vi "程序下载-V1.0.1.vi"() -> ()   [LabVIEW 2013]
uses:
  SxsenderClassLibrary.dll
panel:
  out "x/y":dbl format="%.1f"
  in  "SX文件路径 2":path
  in  "基路径 2":path=path "C:/Program Files/National Instruments/LabVIEW 2013/temp"
  out "添加的路径":path
  out "引用输出":refnum<k24>
  in  "布尔":bool
  in  "停止":bool
  in  "基路径":path=path "C:/Program Files/National Instruments/LabVIEW 2013/temp"
  out "错误输出":errorcluster
  in  "停止":bool
  out "字符串":string
  in  "结果":i32(listbox)=-1
  out "Schedule":u8(slide) scale=0.0..100.0
  in  "Slave NO.":u16(ring) items=["1", "2", "3", "4", "5", "6", "7", "8", "9", "10", "11", "12", "13", "14", "15", "16", "17", "18", "19", "20", "21", "22", "23", "24", "25", "26", "27", "28", "29", "30", ""]
  in  "CAN端口 2":u16(ring)=2 caption="TargetBoard" items=["BCU"=1, "BMU"=2]
  in  "波特率":u16(ring)=500 caption="Baudrate" items=["5Kbps"=5, "10Kbps"=10, "20Kbps"=20, "40Kbps"=40, "50Kbps"=50, "80Kbps"=80, "100Kbps"=100, "125Kbps"=125, "200Kbps"=200, "250Kbps"=250, "400Kbps"=400, "500Kbps"=500, "666Kbps"=666, "800Kbps"=800, "1000Kbps"=1000]
  in  "STOP":bool
  in  "Continue":bool
  in  "START":bool
  in  "SX File Path":path
  in  "CAN端口":u16(ring) caption="CANIndex" items=["0", "1"]
  in  "CAN卡类型":u32(ring)=4 caption="DevType" items=["PCI5121"=1, "PCI9810"=2, "USBCAN1"=3, "USBCAN2"=4, "PCI9820"=5, "PCI5110"=7, "CANLite(mini)"=8, "ISA9620"=9, "ISA5420"=10, "PC104CAN"=11, "DNP9810"=13, "PCI9840B"=14, "PC104C2"=15, "PCI9820I"=16, "pec9920"=18, "USBCAN_E_U"=20, "USBCAN_2E_U"=21]
  in  "设备索引号":u16(ring) caption="DevIndex" items=["0", "1", "2", "3", "4", "5", "6", "7", "8", "9", "10", "11", "12", "13", "14", "15", "16"]
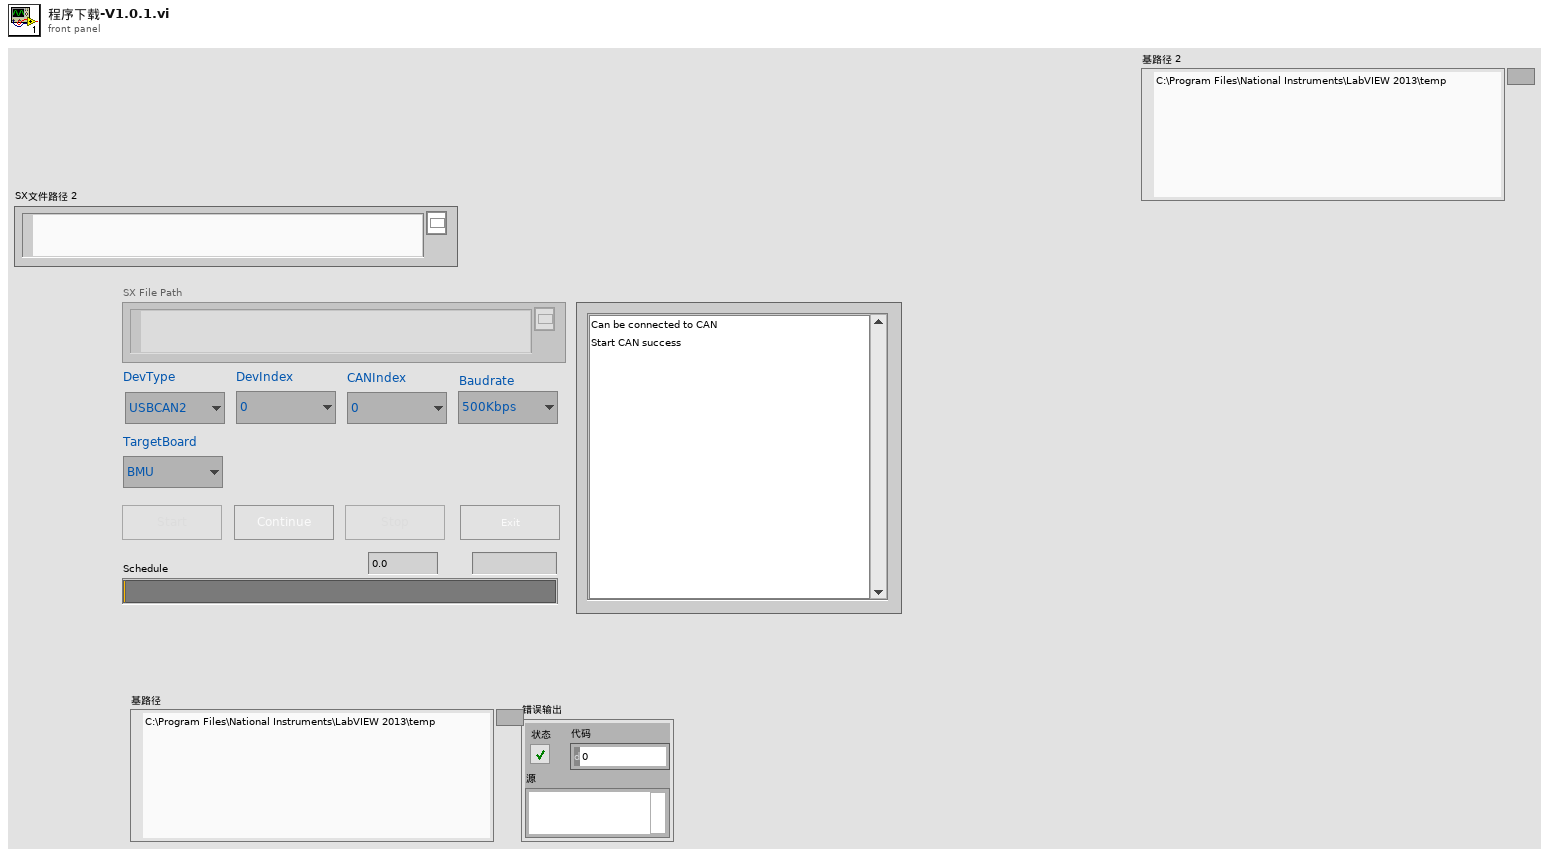
[diagram p1: front panel]
types:
  T1 = enum32{"Invalid", "Standard", "Closed", "Hidden", "Minimized", "Maximized"}
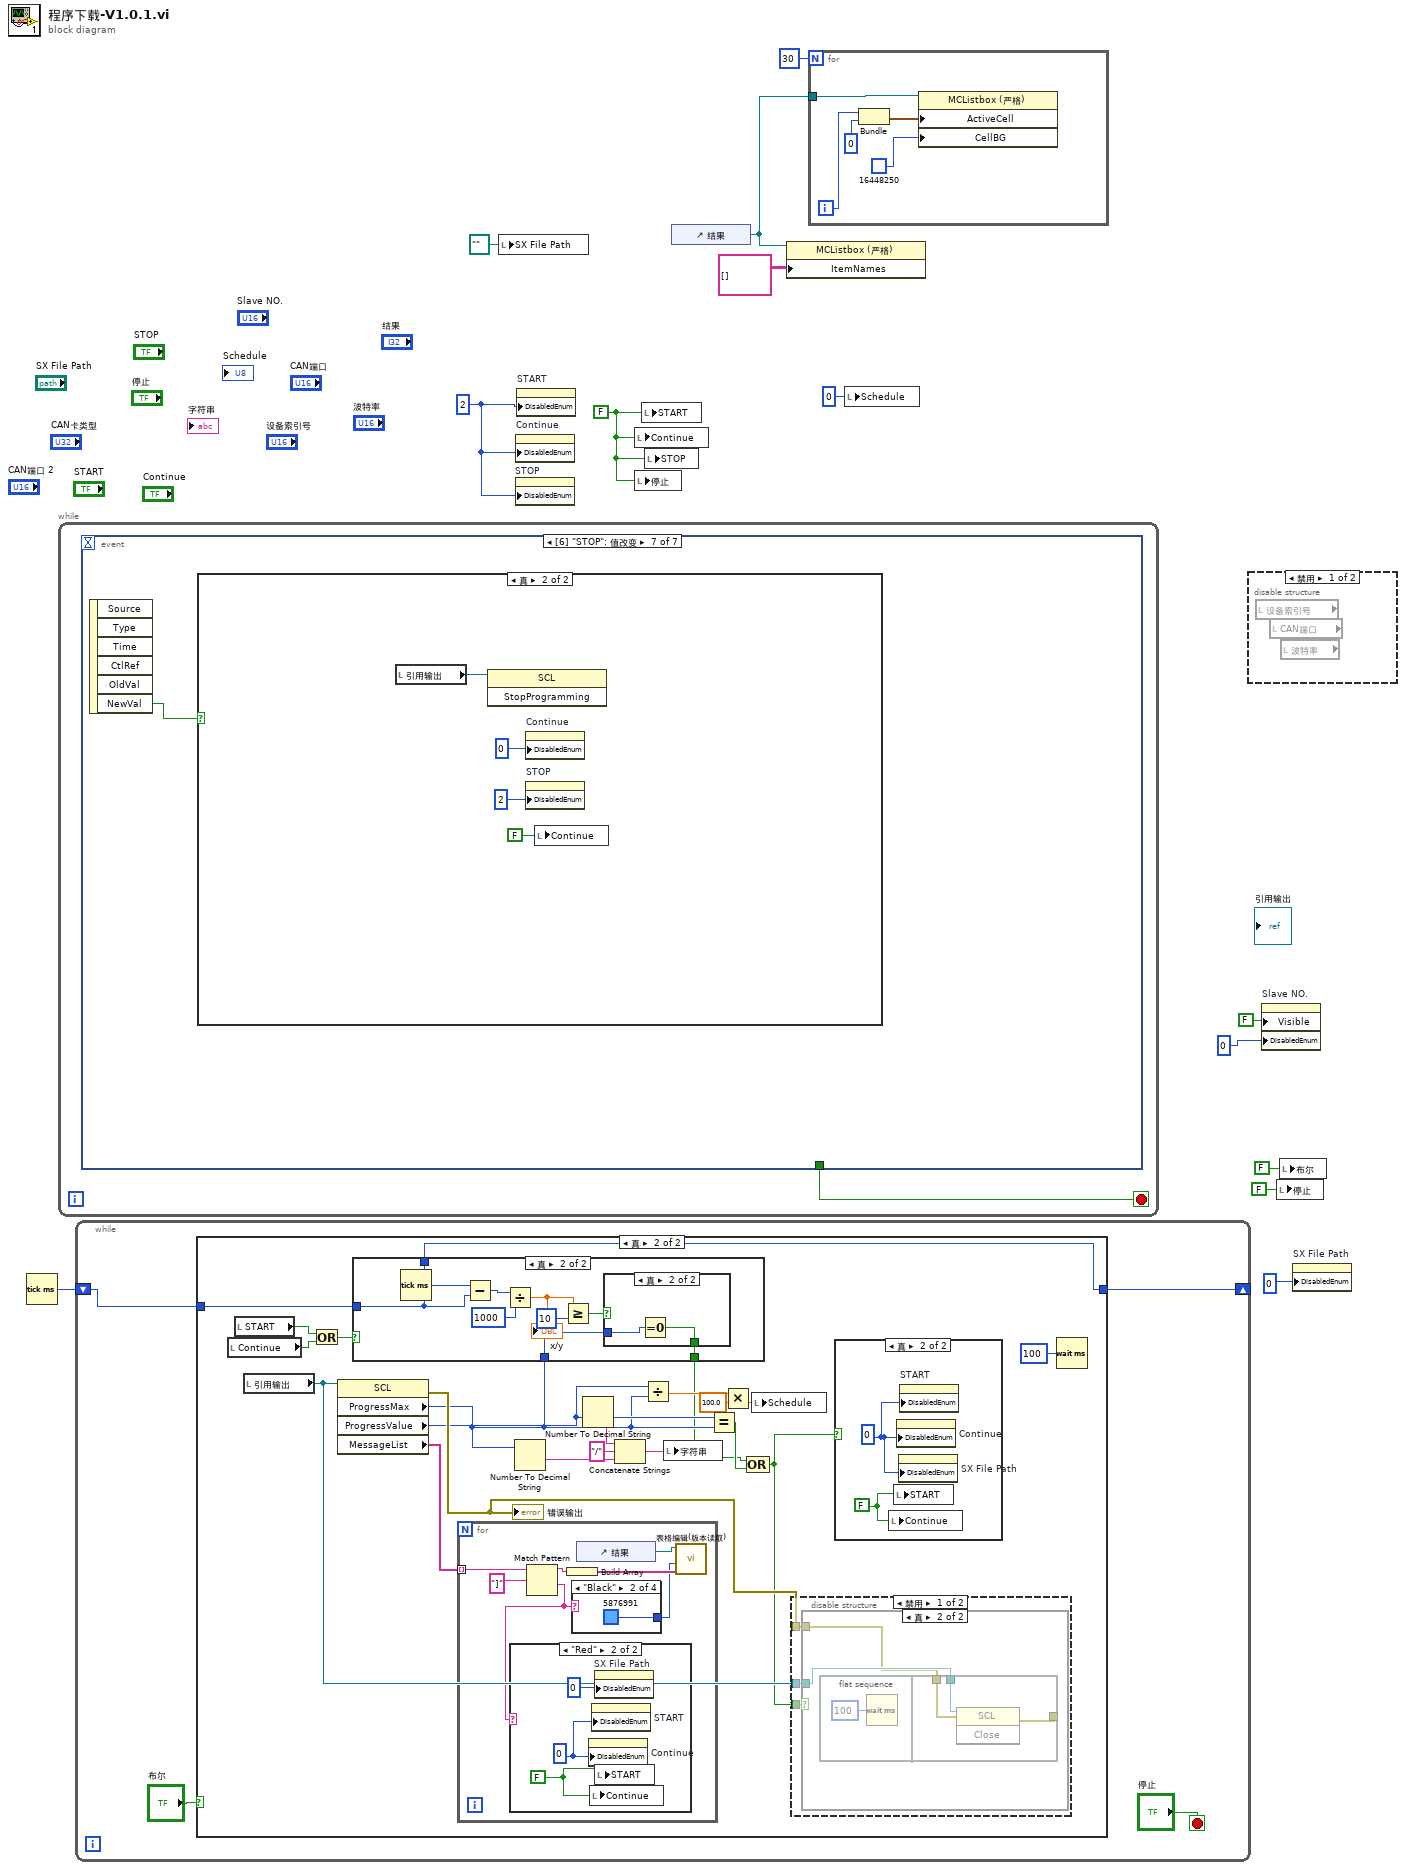
[diagram p0: block diagram]
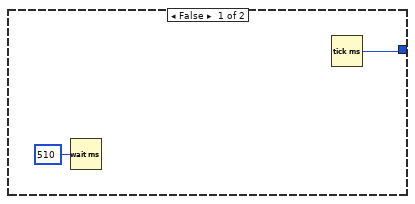
[diagram p3: hidden frame]
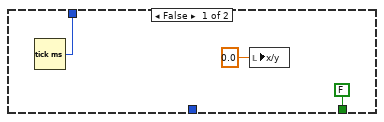
[diagram p4: hidden frame]
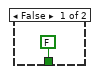
[diagram p5: hidden frame]
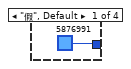
[diagram p10: hidden frame]
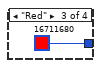
[diagram p11: hidden frame]
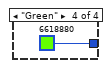
[diagram p12: hidden frame]
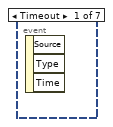
[diagram p13: hidden frame]
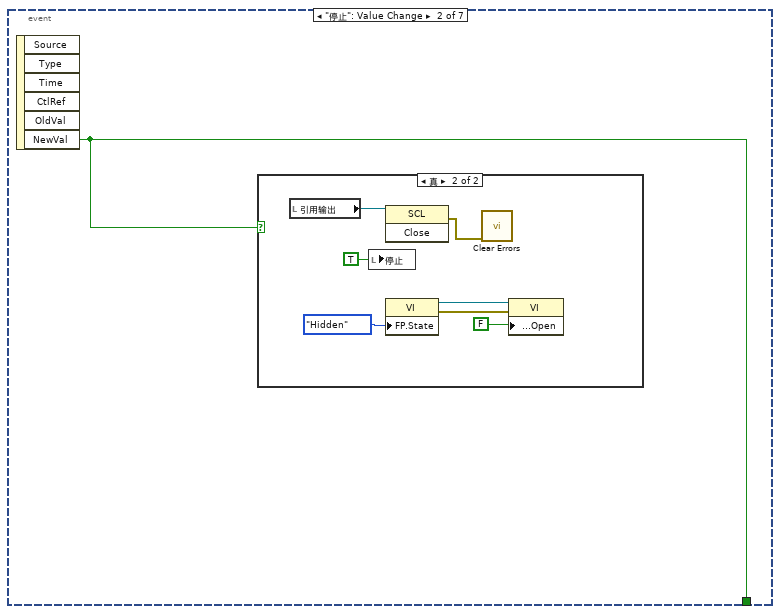
[diagram p14: hidden frame]
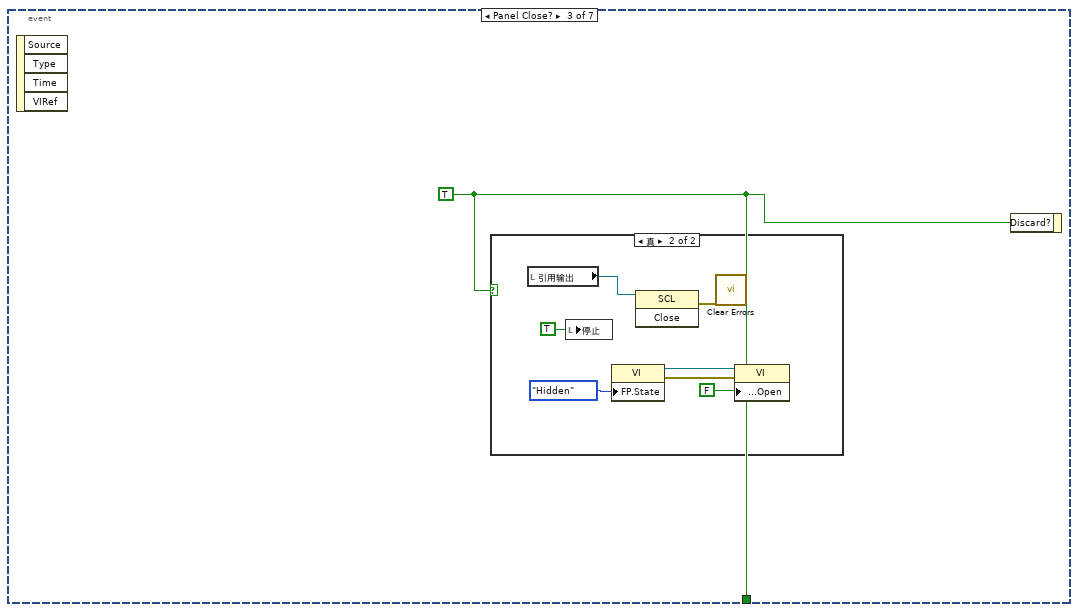
[diagram p16: hidden frame]
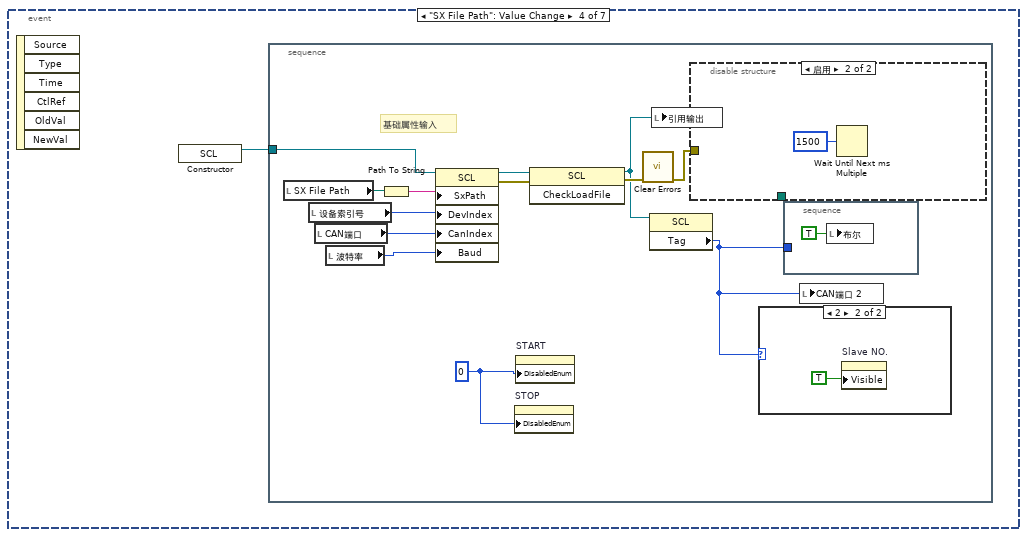
[diagram p18: hidden frame]
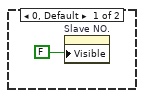
[diagram p19: hidden frame]
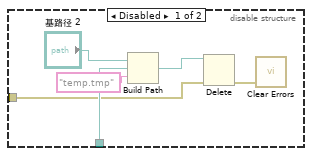
[diagram p20: hidden frame]
diagram:
  w12 = FALSE ("开始刷写")
  w11 = 2
  n1 = Tick Count (ms)() -> (millisecond timer value=w4:u32)
  n2 = while {
    stop <- w14 stop-if-true
    n3 = event shown="[6] \"STOP\": 值改变" {
      selector: _ -> [_ _ _ _ _ _ _]
      dyn-events: _ -> [_ _ _ _ _ _ _]
      timeout: _ -> [_ _ _ _ _ _ _]
      tunnel: [_ w15 w23 _ _ _ _] -> w14
      event Timeout {
        n4 = event-data() -> ()  [unwired: 1 in, 3 out]
      }
      event "停止": Value Change {
        n5 = event-data() -> ("NewVal"=w15:bool)  [unwired: 1 in, 5 out]
        n6 = case shown="真" w15 {
          frame False {
          }
          frame True {
            n7 = local read "引用输出"() -> (w22:refnum<k24>)
            n8 = local write "停止"(TRUE ("停止")) -> ()
            n9 = invoke on="调用节点" class="SCL" method="Close"(reference=w22) -> (error out=w16:errorcluster)  [unwired: 2 in, 2 out]
            n10 = property class="VI"("FP.State"=T1."Hidden" ("前面板窗口:状态")) -> (reference out=w18:refnum<vi>, error out=w17:errorcluster)  [unwired: 2 in]
            n11 = call <vilib>:"Clear Errors.vi"("error in (no error)"=w16) -> ()  [unwired: 6 in, 1 out]
            n12 = property class="VI"(reference=w18, error in=w17, "Front Panel.Open"=FALSE ("前面板窗口:打开")) -> ()  [unwired: 2 out]
          }
        }
      }
      event Panel Close? {
        w23 = TRUE
        n13 = event-data() -> ()  [unwired: 1 in, 4 out]
        n14 = case shown="真" w23 {
          frame False {
          }
          frame True {
            n15 = local read "引用输出"() -> (w30:refnum<k24>)
            n16 = local write "停止"(TRUE ("停止")) -> ()
            n17 = property class="VI"("FP.State"=T1."Hidden" ("前面板窗口:状态")) -> (reference out=w26:refnum<vi>, error out=w25:errorcluster)  [unwired: 2 in]
            n18 = invoke on="调用节点" class="SCL" method="Close"(reference=w30) -> (error out=w24:errorcluster)  [unwired: 2 in, 2 out]
            n19 = call <vilib>:"Clear Errors.vi"("error in (no error)"=w24) -> ()  [unwired: 6 in, 1 out]
            n20 = property class="VI"(reference=w26, error in=w25, "Front Panel.Open"=FALSE ("前面板窗口:打开")) -> ()  [unwired: 2 out]
          }
        }
        n21 = event-data("Discard?"=w23) -> ()  [unwired: 1 in, 1 out]
      }
      event "SX File Path": Value Change {
        n22 = event-data() -> ()  [unwired: 1 in, 6 out]
        n23 = constructor class="SCL"() -> (reference out=w31:refnum<k24>)  [unwired: 3 in, 2 out]
        n24 = stacked-sequence {
          tunnel: w31 -> [w44]
          frame #0 {
            w37 = 0
            # "基础属性输入"
            n25 = local read "SX File Path"() -> (w43:path)
            n26 = local read "设备索引号"() -> (w33:u16)
            n27 = local read "CAN端口"() -> (w32:u16)
            n28 = local read "波特率"() -> (w34:u16)
            n29 = Path To String(path=w43) -> (string=w42:string)
            n30 = property on="属性节点" class="SCL"(reference=w44, "SxPath"=w42, "DevIndex"=w33, "CanIndex"=w32, "Baud"=w34) -> (reference out=w38:refnum<k24>, error out=w41:errorcluster)  [unwired: 1 in]
            n31 = property on="STOP" class="Bool (严格)"("DisabledEnum"=w37) -> ()  [unwired: 2 in, 2 out]
            n32 = property on="START" class="Bool (严格)"("DisabledEnum"=w37) -> ()  [unwired: 2 in, 2 out]
            n33 = invoke on="调用节点" class="SCL" method="CheckLoadFile"(reference=w38, error in=w41) -> (reference out=w36:refnum<k24>, error out=w40:errorcluster)  [unwired: 1 in, 1 out]
            n34 = call <vilib>:"Clear Errors.vi"("error in (no error)"=w40) -> ("error out"=w39:errorcluster)  [unwired: 6 in]
            n35 = property on="属性节点" class="SCL"(reference=w36) -> ("Tag"=w35:u32)  [unwired: 1 in, 2 out]
            n36 = local write "引用输出"(w36) -> ()
            n37 = disable-structure shown="启用" {
              disable-tunnel: [w51 _] -> _
              disable-tunnel: w39 -> [w50 _]
              frame Disabled {
                n38 = Build Path(base path="基路径 2", name or relative path="temp.tmp" ("名称或相对路径")) -> (appended path=w51:path)
                n39 = Delete(path (use dialog)=w51, error in=w50) -> (error out=w49:errorcluster)  [unwired: 3 in, 2 out]
                n40 = call <vilib>:"Clear Errors.vi"("error in (no error)"=w49) -> ()  [unwired: 6 in, 1 out]
              }
              frame Enabled {
                n41 = Wait Until Next ms Multiple(millisecond multiple=u32 1500 ("毫秒倍数")) -> ()  [unwired: 1 out]
              }
            }
            n42 = case shown="2" w35 {
              frame 0, Default {
                n43 = property on="Slave NO." class="Ring (严格)"("Visible"=FALSE ("可见")) -> ()  [unwired: 2 in, 2 out]
              }
              frame 2 {
                n44 = property on="Slave NO." class="Ring (严格)"("Visible"=TRUE ("可见")) -> ()  [unwired: 2 in, 2 out]
              }
            }
            n45 = stacked-sequence {
              tunnel: w35 -> [_]
              frame #0 {
                n46 = local write "布尔"(TRUE ("布尔")) -> ()
              }
            }
            n47 = local write "CAN端口 2"(w35) -> ()
          }
        }
      }
      event "START": Value Change {
        n48 = event-data() -> ("NewVal"=w54:bool)  [unwired: 1 in, 5 out]
        n49 = case shown="真" w54 {
          frame False {
          }
          frame True {
            n50 = stacked-sequence {
              seq-local: [w60 _] -> [_ w70]
              frame #0 {
                # "基础属性输入"
                n51 = local read "引用输出"() -> (w57:refnum<k24>)
                n52 = local read "Slave NO."() -> (w56:u16)
                n53 = Increment(x=w56) -> (x+1=w55:u16)
                n54 = property on="属性节点" class="SCL"(reference=w57, "BmuID"=w55) -> (reference out=w60:refnum<k24>)  [unwired: 1 in, 1 out]
                n55 = call <vilib>:"Clear Errors.vi"() -> ("error out"=w58:errorcluster)  [unwired: 7 in]
                n56 = disable-structure shown="启用" {
                  disable-tunnel: [w64 _] -> w59
                  disable-tunnel: w58 -> [w63 _]
                  frame Disabled {
                    n57 = Build Path(base path="基路径", name or relative path="temp.tmp" ("名称或相对路径")) -> (appended path=w64:path)
                    n58 = Delete(path (use dialog)=w64, error in=w63) -> (error out=w62:errorcluster)  [unwired: 3 in, 2 out]
                    n59 = call <vilib>:"Clear Errors.vi"("error in (no error)"=w62) -> ()  [unwired: 6 in, 1 out]
                  }
                  frame Enabled {
                    n60 = Wait Until Next ms Multiple(millisecond multiple=u32 1500 ("毫秒倍数")) -> ()  [unwired: 1 out]
                  }
                }
                "添加的路径" <- w59
              }
              frame #1 {
                w68 = 2
                n61 = local write "STOP"(FALSE ("终止刷写")) -> ()
                n62 = property on="START" class="Bool (严格)"("DisabledEnum"=w68) -> ()  [unwired: 2 in, 2 out]
                n63 = property on="Continue" class="Bool (严格)"("DisabledEnum"=w68) -> ()  [unwired: 2 in, 2 out]
                n64 = invoke on="调用节点" class="SCL" method="StartProgramming"(reference=w70) -> (reference out=w71:refnum<k24>)  [unwired: 2 in, 2 out]
                n65 = property on="SX File Path" class="Path"("DisabledEnum"=2) -> ()  [unwired: 2 in, 2 out]
                n66 = local write "引用输出"(w71) -> ()
              }
            }
          }
        }
      }
      event "Continue": Value Change {
        n67 = event-data() -> ("NewVal"=w72:bool)  [unwired: 1 in, 5 out]
        n68 = case shown="真" w72 {
          frame False {
          }
          frame True {
            n69 = local read "引用输出"() -> (w77:refnum<k24>)
            n70 = invoke on="调用节点" class="SCL" method="Continueprogramming"(reference=w77) -> (reference out=w76:refnum<k24>)  [unwired: 2 in, 2 out]
            n71 = property on="Continue" class="Bool (严格)"("DisabledEnum"=2) -> ()  [unwired: 2 in, 2 out]
            n72 = property on="STOP" class="Bool (严格)"("DisabledEnum"=0) -> ()  [unwired: 2 in, 2 out]
            n73 = local write "STOP"(FALSE ("终止刷写")) -> ()
            n74 = local write "引用输出"(w76) -> ()
          }
        }
      }
      event "STOP": Value Change {
        n75 = event-data() -> ("NewVal"=w78:bool)  [unwired: 1 in, 5 out]
        n76 = case shown="真" w78 {
          frame False {
          }
          frame True {
            n77 = local read "引用输出"() -> (w81:refnum<k24>)
            n78 = invoke on="调用节点" class="SCL" method="StopProgramming"(reference=w81) -> ()  [unwired: 2 in, 3 out]
            n79 = property on="Continue" class="Bool (严格)"("DisabledEnum"=0) -> ()  [unwired: 2 in, 2 out]
            n80 = property on="STOP" class="Bool (严格)"("DisabledEnum"=2) -> ()  [unwired: 2 in, 2 out]
            n81 = local write "Continue"(FALSE ("Continue")) -> ()
          }
        }
      }
    }
  }
  n82 = while {
    shift-right: [w84] -> _
    shift-left: w4 -> [w83]
    stop <- "停止" stop-if-true
    n83 = case shown="真" "布尔" {
      tunnel: [w87 w89] -> w84
      tunnel: w83 -> [_ w94]
      frame False {
        n84 = Wait (ms)(milliseconds to wait=u32 510 ("等待时间（毫秒）")) -> ()  [unwired: 1 out]
        n85 = Tick Count (ms)() -> (millisecond timer value=w87:u32)
      }
      frame True {
        n86 = local read "Continue"() -> (w91:bool)
        n87 = local read "START"() -> (w92:bool)
        n88 = local read "引用输出"() -> (w101:refnum<k24>)
        n89 = Or(x=w92, y=w91) -> (x .or. y?=w90:bool)
        n90 = property on="属性节点" class="SCL"(reference=w101) -> (error out=w99:errorcluster, "ProgressMax"=w96:u32, "ProgressValue"=w98:u32, "MessageList"=w100:string[])  [unwired: 1 in, 1 out]
        "错误输出" <- w99
        n91 = case shown="真" w90 {
          tunnel: w96 -> [_ w115]
          tunnel: [FALSE w114] -> w95
          tunnel: w94 -> [_ w113]
          tunnel: [w111 w113] -> w89
          frame False {
            n92 = Tick Count (ms)() -> (millisecond timer value=w111:u32)
            n93 = local write "x/y"(0.0 ("x/y")) -> ()
          }
          frame True {
            n94 = Tick Count (ms)() -> (millisecond timer value=w121:u32)
            n95 = Subtract(x=w121, y=w113) -> (x-y=w120:u32)
            n96 = Divide(x=w120, y=u32 1000) -> (x/y=w118:dbl)
            "x/y" <- w118
            n97 = Greater Or Equal?(x=w118, y=u32 10) -> (x >= y?=w116:bool)
            n98 = case shown="真" w116 {
              tunnel: w115 -> [_ w124]
              tunnel: [FALSE w123] -> w114
              frame False {
              }
              frame True {
                n99 = Equal To 0?(x=w124) -> (x = 0?=w123:bool)
              }
            }
          }
        }
        n100 = for {
          tunnel: w100 -> [w137] mode=indexing
          n101 = Match Pattern(string=w137, regular expression="]") -> (before substring=w140:string, after substring=w136:string)  [unwired: 1 in, 2 out]
          n102 = case shown="\"Red\"" w136 {
            frame "假", Default {
            }
            frame "Red" {
              w144 = FALSE
              w145 = 0
              n103 = property on="Continue" class="Bool (严格)"("DisabledEnum"=w145) -> ()  [unwired: 2 in, 2 out]
              n104 = local write "Continue"(w144) -> ()
              n105 = property on="START" class="Bool (严格)"("DisabledEnum"=w145) -> ()  [unwired: 2 in, 2 out]
              n106 = property on="SX File Path" class="Path"("DisabledEnum"=0) -> ()  [unwired: 2 in, 2 out]
              n107 = local write "START"(w144) -> ()
            }
          }
          n108 = Build Array(w140) -> (w139:string[])
          n109 = case shown="\"Black\"" w136 {
            tunnel: [u32 5876991 u32 5876991 u32 16711680 u32 6618880] -> w138
            frame "假", Default {
            }
            frame "Black" {
            }
            frame "Red" {
            }
            frame "Green" {
            }
          }
          n110 = control-ref of="结果"() -> (w142:refnum<vi>)
          n111 = call "表格编辑(版本读取).vi"("新元素/子数组"=w139, "活动单元格:单元格背景色"=w138, "MCListbox引用句柄"=w142) -> ()  [unwired: 9 in]
        }
        n112 = Number To Decimal String(number=w96) -> (decimal integer string=w105:string)  [unwired: 1 in]
        n113 = Number To Decimal String(number=w98) -> (decimal integer string=w104:string)  [unwired: 1 in]
        n114 = Concatenate Strings(w104, "/" ("字符串"), w105) -> (w102:string)
        n115 = Divide(x=w98, y=w96) -> (x/y=w108:dbl)
        n116 = local write "字符串"(w102) -> ()
        n117 = Equal?(x=w98, y=w96) -> (x = y?=w109:bool)
        n118 = Multiply(x=w108, y=100.0) -> (x*y=w106:dbl)
        n119 = Compound Arithmetic op=OR(w95, w109) -> (w93:bool)
        n120 = local write "Schedule"(w106) -> ()
        n121 = disable-structure shown="禁用" {
          disable-tunnel: w93 -> [w129 _]
          disable-tunnel: w101 -> [w128 _]
          disable-tunnel: w99 -> [w127 _]
          frame Disabled {
            n122 = case shown="真" w129 {
              tunnel: w128 -> [_ w131]
              tunnel: w127 -> [_ w130]
              frame False {
              }
              frame True {
                n123 = flat-sequence {
                  tunnel: w130 -> [w134]
                  tunnel: [w135] -> _
                  tunnel: w131 -> [w133]
                  frame #0 {
                    n124 = Wait (ms)(milliseconds to wait=u32 100 ("等待时间（毫秒）")) -> ()  [unwired: 1 out]
                  }
                  frame #1 {
                    n125 = invoke class="SCL" method="Close"(reference=w133, error in=w134) -> (error out=w135:errorcluster)  [unwired: 1 in, 2 out]
                  }
                }
              }
            }
          }
          frame Enabled {
          }
        }
        n126 = case shown="真" w93 {
          frame False {
          }
          frame True {
            w126 = FALSE
            w125 = 0
            n127 = local write "Continue"(w126) -> ()
            n128 = local write "START"(w126) -> ()
            n129 = property on="Continue" class="Bool (严格)"("DisabledEnum"=w125) -> ()  [unwired: 2 in, 2 out]
            n130 = property on="SX File Path" class="Path"("DisabledEnum"=w125) -> ()  [unwired: 2 in, 2 out]
            n131 = property on="START" class="Bool (严格)"("DisabledEnum"=w125) -> ()  [unwired: 2 in, 2 out]
          }
        }
        n132 = Wait (ms)(milliseconds to wait=u32 100 ("等待时间（毫秒）")) -> ()  [unwired: 1 out]
      }
    }
  }
  n133 = local write "SX File Path"(path "" ("SX文件路径")) -> ()
  n134 = property on="Continue" class="Bool (严格)"("DisabledEnum"=w11) -> ()  [unwired: 2 in, 2 out]
  n135 = property on="STOP" class="Bool (严格)"("DisabledEnum"=w11) -> ()  [unwired: 2 in, 2 out]
  n136 = property on="START" class="Bool (严格)"("DisabledEnum"=w11) -> ()  [unwired: 2 in, 2 out]
  n137 = local write "Continue"(w12) -> ()
  n138 = local write "停止"(w12) -> ()
  n139 = local write "START"(w12) -> ()
  n140 = local write "STOP"(w12) -> ()
  n141 = control-ref of="结果"() -> (w6:refnum<vi>)
  n142 = property class="MCListbox (严格)"(reference=w6, "ItemNames"=string[][] [] ("项名")) -> ()  [unwired: 1 in, 2 out]
  n143 = for {
    N: 30 -> [_]
    tunnel: w6 -> [w154]
    i -> [w151]
    n144 = Bundle(w151, 0) -> (w153:cluster{i32, i32})  [unwired: 1 out]
    n145 = property class="MCListbox (严格)"(reference=w154, "ActiveCell"=w153, "CellBG"=u32 16448250) -> ()  [unwired: 1 in, 2 out]
  }
  n146 = local write "Schedule"(u8 0 ("刷写进度")) -> ()
  n147 = disable-structure shown="禁用" {
    frame Disabled {
      n148 = local read "设备索引号"() -> ()  [unwired: 1 out]
      n149 = local read "CAN端口"() -> ()  [unwired: 1 out]
      n150 = local read "波特率"() -> ()  [unwired: 1 out]
    }
    frame Enabled {
    }
  }
  n151 = property on="Slave NO." class="Ring (严格)"("Visible"=FALSE ("可见"), "DisabledEnum"=0) -> ()  [unwired: 2 in, 2 out]
  n152 = local write "停止"(FALSE ("停止")) -> ()
  n153 = local write "布尔"(FALSE ("布尔")) -> ()
  n154 = property on="SX File Path" class="Path"("DisabledEnum"=0) -> ()  [unwired: 2 in, 2 out]
